vi "Generate Discovery Client.vi"(8 "error in (no error)":errorcluster) -> (0 "error out":errorcluster)   [LabVIEW 2020, in "MeasurementLink Proto Builds.lvlib"]
uses:
  MeasurementLink Proto Builds.lvlib
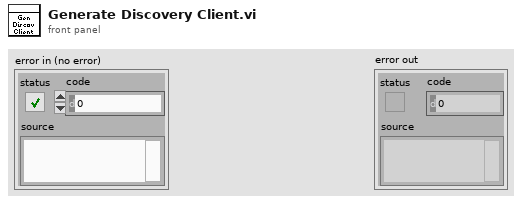
[diagram p1: front panel]
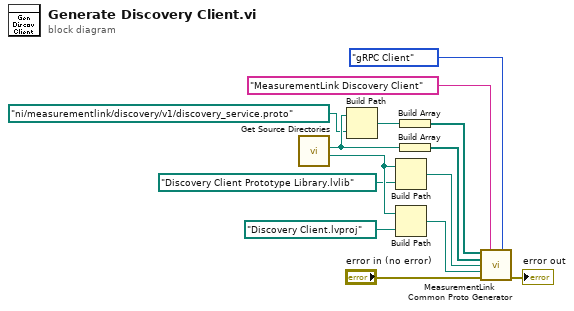
[diagram p0: block diagram]
diagram:
  n1 = call "Get Source Directories.vi"() -> ("Runtime Dir"=w6:path, "Protos Dir"=w2:path)  [unwired: 9 in, 1 out]
  n2 = Build Path(base path=w2, name or relative path=path "ni/measurementlink/discovery/v1/discovery_service.proto" ("Proto File Path")) -> (appended path=w3:path)
  n3 = Build Path(base path=w6, name or relative path=path "Discovery Client Prototype Library.lvlib") -> (appended path=w4:path)
  n4 = Build Path(base path=w6, name or relative path=path "Discovery Client.lvproj" ("Target Project")) -> (appended path=w7:path)
  n5 = Build Array(w3) -> (w9:path[])
  n6 = Build Array(w2) -> (w10:path[])
  n7 = call "MeasurementLink Common Proto Generator.vi"("Proto File Path"=w9, "Generated Library Full Name"="MeasurementLink Discovery Client" ("Generated Library Name"), "Generate"=enum16{"gRPC Server", "gRPC Client", "Both"}."gRPC Client", "Import Paths"=w10, "Prototype Library"=w4, "Target Project"=w7, "error in (no error)"="error in (no error)") -> ("error out"=→"error out":errorcluster)  [unwired: 8 in]
